vi "Read Scanner UDP Handle.vi"(8 "error in (no error)":errorcluster, 11 "PF_API in":refnum<class "PF_API.lvclass">) -> (0 "error out":errorcluster, 2 "Scanner UDP Handle":string, 3 "PF_API out":refnum<class "PF_API.lvclass">)   [LabVIEW 2019, in "PF_API.lvclass"]
uses:
  PF_API.lvclass
  PF_API.lvclass/PF_API.ctl
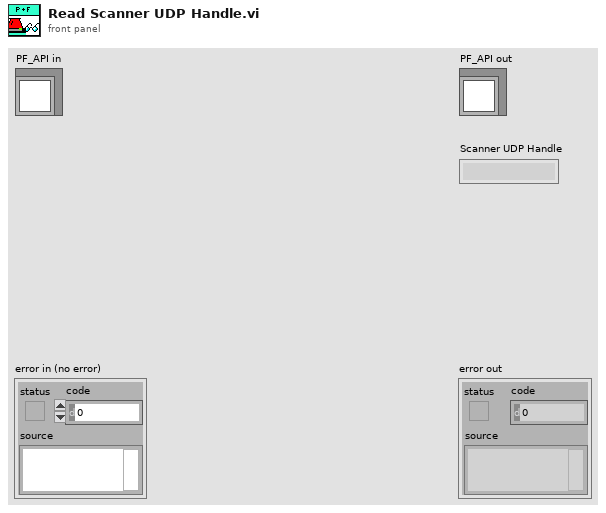
[diagram p1: front panel]
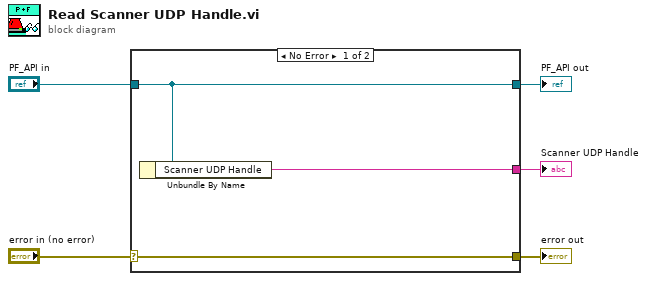
[diagram p0: block diagram]
diagram:
  n1 = case shown="No Error" "error in (no error)" {
    selector: "error in (no error)" -> [w8 w9]
    tunnel: [w8 w9] -> w4
    tunnel: [w7 w10] -> w2
    tunnel: "PF_API in" -> [w7 w10]
    tunnel: [w6 _] -> w1
    frame No Error {
      n2 = Unbundle By Name(w7) -> ("Scanner UDP Handle"=w6:string)
    }
    frame Error {
    }
  }
  "error out" <- w4
  "PF_API out" <- w2
  "Scanner UDP Handle" <- w1
